vi "Create.vi"(8 "error in (no error)":errorcluster, 9 "Image Size":T1, 11 "Camera Parameters in":T2) -> (0 "error out":errorcluster, 3 "New ImageDistorter":refnum<class "ImageDistorter.lvclass">)   [LabVIEW 2020, in "g_ar_toolkit.image.lvlib" / "ImageDistorter.lvclass"]
uses:
  ImageDistorter.lvclass
  g_ar_toolkit.common/Camera Parameters.ctl
  g_ar_toolkit.common/Camera Matrix.ctl
  g_ar_toolkit.common/Camera Distortion Coefficients.ctl
  g_ar_toolkit.common/Image Size (Integer).ctl
  ImageDistorter.lvclass/ImageDistorter.ctl
  g_ar_toolkit.common/g_ar_toolkit.common.lvlib
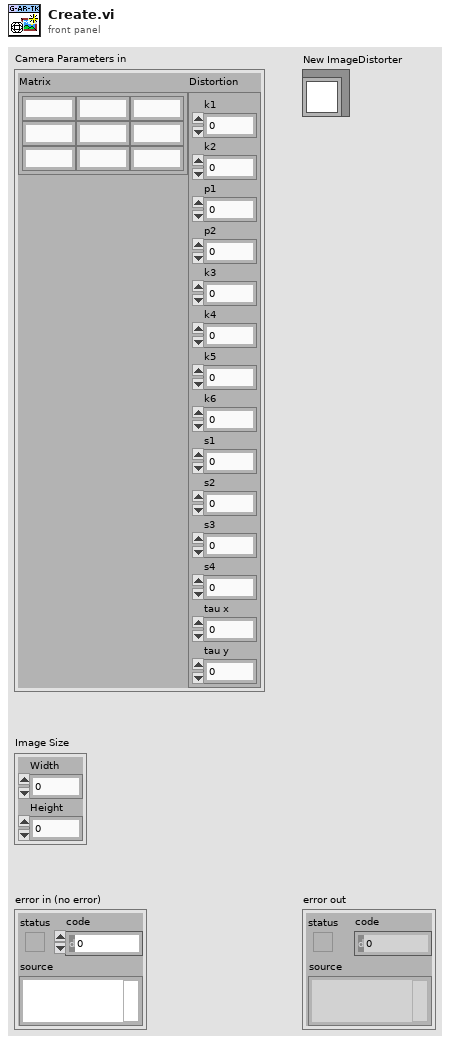
[diagram p1: front panel]
types:
  T1 = typedef "g_ar_toolkit.common.lvlib/Image Size (Integer).ctl" = cluster{"Width":u16, "Height":u16}
  T2 = typedef "g_ar_toolkit.common.lvlib/Camera Parameters.ctl" = cluster{"Matrix":T3, "Distortion":T4}
  T3 = typedef "g_ar_toolkit.common.lvlib/Camera Matrix.ctl" = cluster{"m 0,0":dbl, "m 0,1":dbl, "m 0,2":dbl, "m 1,0":dbl, "m 1,1":dbl, "m 1,2":dbl, "m 2,0":dbl, "m 2,1":dbl, "m 2,2":dbl}
  T4 = typedef "g_ar_toolkit.common.lvlib/Camera Distortion Coefficients.ctl" = cluster{"k1":dbl, "k2":dbl, "p1":dbl, "p2":dbl, "k3":dbl, "k4":dbl, "k5":dbl, "k6":dbl, "s1":dbl, "s2":dbl, "s3":dbl, "s4":dbl, "tau x":dbl, "tau y":dbl}
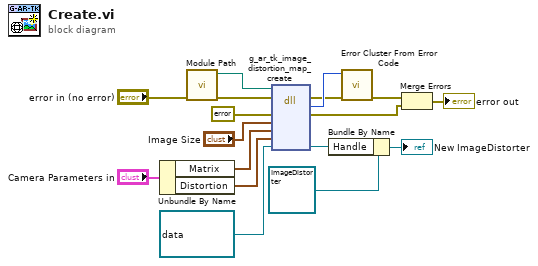
[diagram p0: block diagram]
diagram:
  n1 = Unbundle By Name("Camera Parameters in") -> ("Matrix"=w7:T3, "Distortion"=w6:T4)
  n2 = call "Module Path.vi"("error in (no error)"="error in (no error)") -> ("error out"=w12:errorcluster, "Path"=w11:path)  [unwired: 9 in]
  n3 = dll-call lib="C:/serenial/libraries/g-augmented-reality-toolkit/LabVIEW/g_ar_toolkit.common/bin/g_ar_toolkit.1.32.dll" fn="g_ar_tk_image_distortion_map_create" ("g_ar_toolkit.*.*:g_ar_tk_image_add_weighted")(path in=w11, error in=w12, "error_cluster"=errorcluster {"status"=FALSE, "code"=0, "source"=""} ("error constant"), "size"="Image Size", "camera_matrix"=w7, "distortion_param"=w6, "EDVR"=refnum<data-value> refnum) -> (error out=w13:errorcluster, "MgErr"=w14:i32, "error_cluster"=w17:errorcluster, "EDVR"=w2:refnum<data-value>)  [unwired: 4 in, 1 out]
  n4 = Bundle By Name(cluster=refnum<class "ImageDistorter.lvclass"> refnum ("ImageRectifier out"), "Handle"=w2) -> (→"New ImageDistorter":refnum<class "ImageDistorter.lvclass">)
  n5 = call <vilib>:"Error Cluster From Error Code.vi"("error in (no error)"=w13, "error code (0)"=w14) -> ("error out"=w15:errorcluster)  [unwired: 7 in]
  n6 = Merge Errors(w15, w17) -> (→"error out":errorcluster)
